vi "Load.vi"(8 "error in (no error)":errorcluster, 10 "File":path, 11 "MusicFile In":refnum<class "MusicFile.lvclass">) -> (0 "error out":errorcluster, 3 "MusicFile Out":refnum<class "MusicFile.lvclass">)   [LabVIEW 2015, in "MusicFile.lvclass"]
uses:
  MusicFile.lvclass
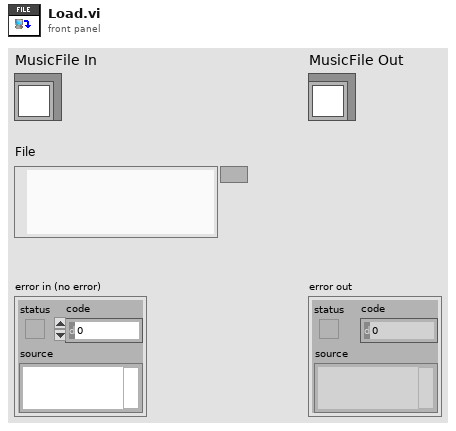
[diagram p1: front panel]
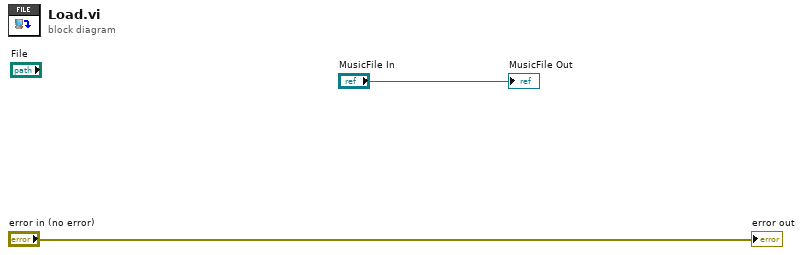
[diagram p0: block diagram]
diagram:
  "error out" <- "error in (no error)"
  "MusicFile Out" <- "MusicFile In"
